vi "Start AI.vi"(6 "error in (no error)":errorcluster, 9 "DAQmx in":refnum<class "DAQmx.lvclass">) -> (0 "error out":errorcluster, 3 "DAQmx out":refnum<class "DAQmx.lvclass">)   [LabVIEW 2019, in "DAQmx.lvclass"]
uses:
  DAQmx.lvclass
  DAQmx.lvclass/DAQmx.ctl
  <vilib>/DAQmx/read.llb/DAQmx Read (Analog 1D Wfm NChan NSamp).vi
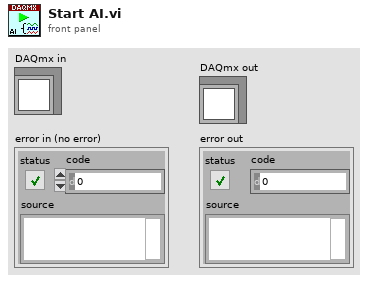
[diagram p1: front panel]
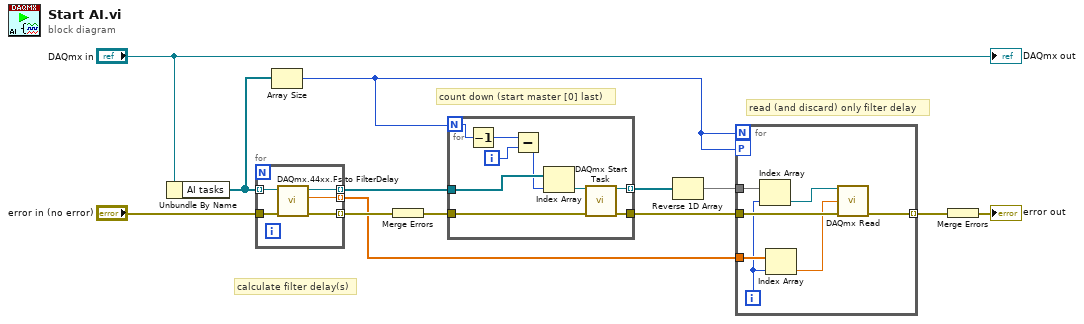
[diagram p0: block diagram]
diagram:
  # "read (and discard) only filter delay"
  # "calculate filter delay(s)"
  # "count down (start master [0] last)"
  n1 = Unbundle By Name("DAQmx in") -> ("AI tasks"=w2:refnum<k21>[])
  n2 = for {
    tunnel: w2 -> [w18] mode=indexing
    tunnel: [w17] -> w11 mode=indexing
    tunnel: [w16] -> w3 mode=indexing
    tunnel: [w15] -> w9 mode=indexing
    tunnel: "error in (no error)" -> [w14]
    n3 = call "DAQmx.44xx.Fs to FilterDelay.vi"("error in (no error)"=w14, "Refnum in"=w18) -> ("error out"=w15:errorcluster, "Filter Delay (samples)"=w16:dbl, "Refnum out"=w17:refnum<k21>)  [unwired: 7 in]
  }
  n4 = Array Size(array=w2) -> (size(s)=w1:i32)
  n5 = Merge Errors(w9) -> (w8:errorcluster)
  n6 = for {
    N: w1 -> [w23]
    tunnel: w8 -> [w27]
    tunnel: [w26] -> w7
    tunnel: w11 -> [w24]
    tunnel: [w19] -> w6 mode=indexing
    i -> [w22]
    n7 = Decrement(x=w23) -> (x-1=w20:i32)
    n8 = Subtract(x=w20, y=w22) -> (x-y=w21:i32)
    n9 = Index Array(array=w24, index=w21) -> (element=w25:refnum<k21>)
    n10 = call <vilib>:"DAQmx Start Task.vi"("task/channels in"=w25, "error in"=w27) -> ("task out"=w19:refnum<k21>, "error out"=w26:errorcluster)  [unwired: 12 in]
  }
  n11 = Reverse 1D Array(array=w6) -> (reversed array=w5:refnum<k21>[])
  n12 = for {
    N: w1 -> [_]
    tunnel: w3 -> [w31]
    tunnel: w5 -> [w32]
    workers-P: w1 -> [_]
    tunnel: w7 -> [w34]
    tunnel: [w33] -> w4 mode=indexing
    i -> [w30]
    n13 = Index Array(array=w32, index=w30) -> (element=w29:refnum<k21>)
    n14 = Index Array(array=w31, index=w30) -> (element=w28:dbl)
    n15 = call-poly <vilib>:"DAQmx Read.vi"("task/channels in"=w29, "number of samples per channel"=w28, "error in"=w34) -> ("error out"=w33:errorcluster)  [unwired: 10 in, 2 out]
  }
  n16 = Merge Errors(w4) -> (→"error out":errorcluster)
  "DAQmx out" <- "DAQmx in"
